vi "Fille Encode.vi"(8 "error in":errorcluster, 11 "Original File":path) -> (2 "string out":string, 10 "Original Data":string)   [LabVIEW 2020]
uses:
  <vilib>/Utility/file.llb/Write Delimited Spreadsheet (string).vi
  <vilib>/Utility/file.llb/Read Delimited Spreadsheet (string).vi
panel:
  out "array":string[][](array[string])
  out "error out":errorcluster
  # "ENCODE"
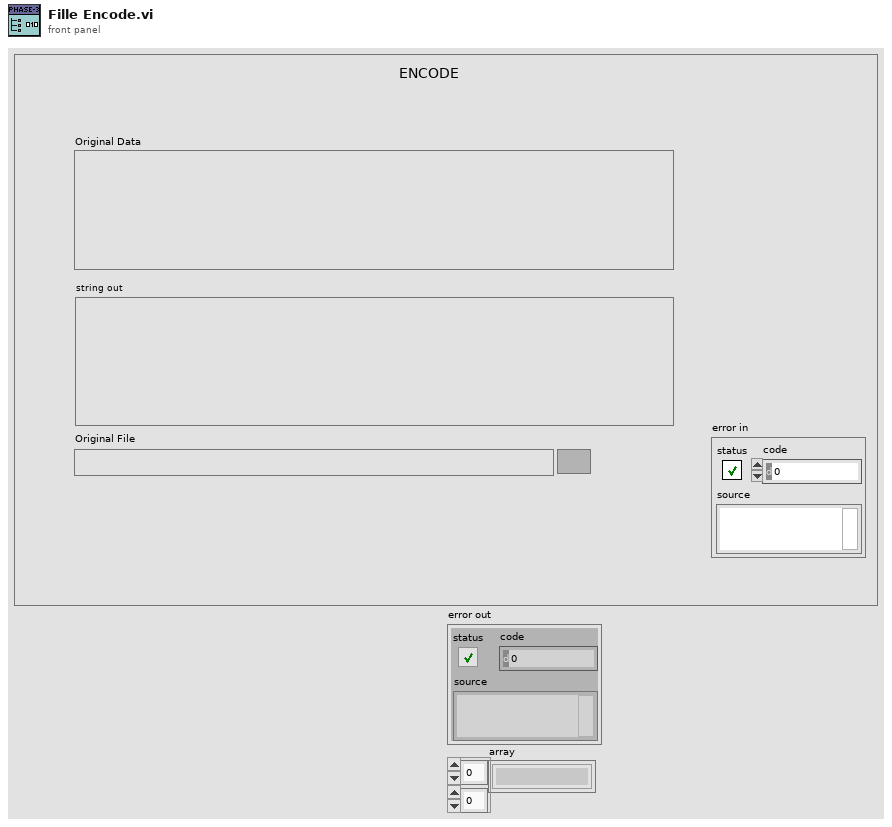
[diagram p1: front panel]
types:
  T1 = cluster{"unsigned byte array[0]":u8, "unsigned byte array[1]":u8, "unsigned byte array[2]":u8}
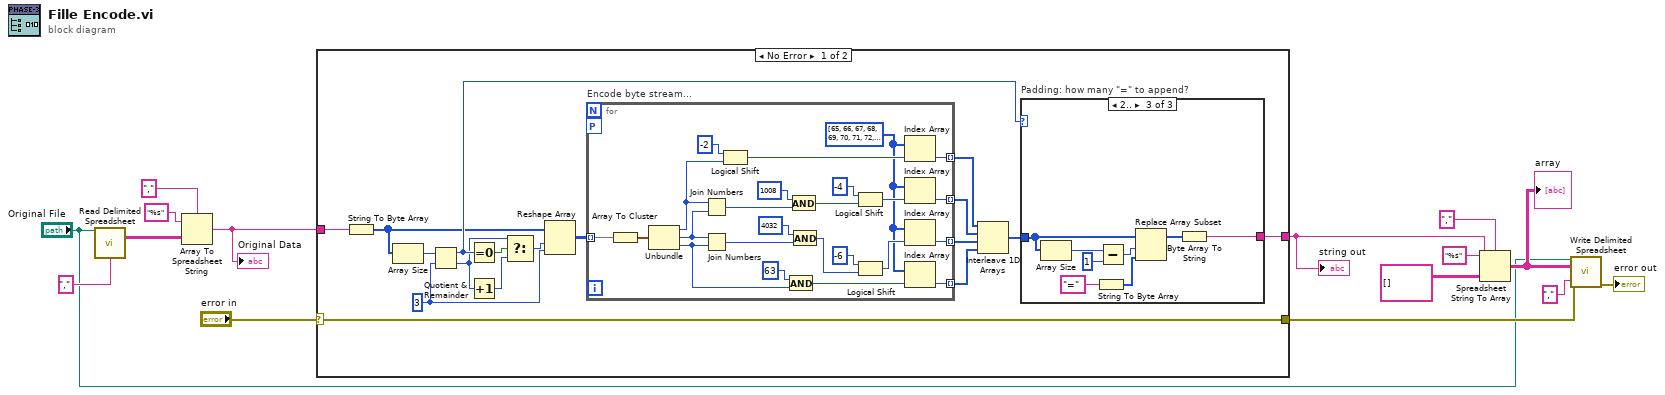
[diagram p0: block diagram]
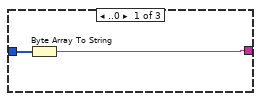
[diagram p2: hidden frame]
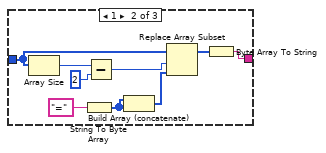
[diagram p3: hidden frame]
diagram:
  n1 = call-poly <vilib>:"Read Delimited Spreadsheet.vi"("file path (dialog if empty)"="Original File", "delimiter (\\t)"="," ("delimiter (\\t)")) -> ("all rows"=w13:string[][])  [unwired: 8 in, 5 out]
  n2 = Array To Spreadsheet String(delimiter (Tab)=",", array=w13, 3:"%s" ("format string")) -> (spreadsheet string=w9:string)
  "Original Data" <- w9
  n3 = case shown="No Error" "error in" {
    selector: "error in" -> [w16 w77]
    tunnel: w9 -> [w19 w76]
    tunnel: [w16 w77] -> w3
    tunnel: [w18 w76] -> w14
    frame No Error {
      w22 = 3 ("y")
      n4 = String To Byte Array(string=w19) -> (unsigned byte array=w23:u8[])
      n5 = Array Size(array=w23) -> (size(s)=w17:i32)
      n6 = Quotient & Remainder(x=w17, y=w22) -> (x-y*floor(x/y)=w31:i32, floor(x/y)=w25:i32)
      n7 = Equal To 0?(x=w31) -> (x = 0?=w32:bool)
      n8 = Increment(x=w25) -> (x+1=w26:i32)
      n9 = Select(t=w25, s=w32, f=w26) -> (s? t:f=w21:i32)
      n10 = Reshape Array(w23, w21, w22) -> (w20:u8[][])
      n11 = for "Encode byte stream..." {
        tunnel: [w35] -> w27 mode=indexing
        tunnel: [w36] -> w28 mode=indexing
        tunnel: [w37] -> w29 mode=indexing
        tunnel: [w38] -> w30 mode=indexing
        workers-P: _ -> [_]
        tunnel: w20 -> [w33] mode=indexing
        w34 = u8[] [65, 66, 67, 68, 69, 70, 71, 72, 73, 74, 75, 76, 77, 78, 79, 80, 81, 82, 83, 84, 85, 86, 87, 88, 89, 90, 97, 98, 99, 100, 101, 102, 103, 104, 105, 106, 107, 108, 109, 110, 111, 112, 113, 114, 115, 116, 117, 118, 119, 120, 121, 122, 48, 49, 50, 51, 52, 53, 54, 55, 56, 57, 43, 47] ("unsigned byte array")
        n12 = Array To Cluster(array=w33) -> (cluster=w56:T1)
        n13 = Unbundle(w56) -> ("unsigned byte array[0]"=w45:u8, "unsigned byte array[1]"=w50:u8, "unsigned byte array[2]"=w44:u8)
        n14 = Join Numbers(hi=w45, lo=w50) -> ((hi.lo)=w54:u16)
        n15 = Join Numbers(hi=w50, lo=w44) -> ((hi.lo)=w49:u16)
        n16 = Logical Shift(y=i8 -2, x=w45) -> (x << y=w42:u8)
        n17 = And(x=u8 63, y=w44) -> (x .and. y?=w39:u8)
        n18 = And(x=u16 1008, y=w54) -> (x .and. y?=w52:u16)
        n19 = And(x=u16 4032, y=w49) -> (x .and. y?=w47:u16)
        n20 = Logical Shift(y=i8 -4, x=w52) -> (x << y=w41:u16)
        n21 = Logical Shift(y=i8 -6, x=w47) -> (x << y=w40:u16)
        n22 = Index Array(array=w34, index=w42) -> (element=w38:u8)
        n23 = Index Array(array=w34, index=w41) -> (element=w37:u8)
        n24 = Index Array(array=w34, index=w40) -> (element=w36:u8)
        n25 = Index Array(array=w34, index=w39) -> (element=w35:u8)
      }
      n26 = Interleave 1D Arrays(w30, w29, w28, w27) -> (w24:u8[])
      n27 = case "Padding: how many \"=\" to append?" shown="2.." w31 {
        tunnel: [w57 w64 w72] -> w18
        tunnel: w24 -> [w58 w62 w70]
        frame ..0 {
          n28 = Byte Array To String(unsigned byte array=w58) -> (string=w57:string)
        }
        frame 1 {
          n29 = Array Size(array=w62) -> (size(s)=w63:i32)
          n30 = String To Byte Array(string="=") -> (unsigned byte array=w60:u8[])
          n31 = Subtract(x=w63, y=2) -> (x-y=w66:i32)
          n32 = Build Array (concatenate)(w60, w60) -> (w59:u8[])
          n33 = Replace Array Subset(array=w62, new element=w59, index=w66) -> (w65:u8[])
          n34 = Byte Array To String(unsigned byte array=w65) -> (string=w64:string)
        }
        frame 2.. {
          n35 = Array Size(array=w70) -> (size(s)=w71:i32)
          n36 = String To Byte Array(string="=") -> (unsigned byte array=w68:u8[])
          n37 = Subtract(x=w71, y=1) -> (x-y=w74:i32)
          n38 = Replace Array Subset(array=w70, new element=w68, index=w74) -> (w73:u8[])
          n39 = Byte Array To String(unsigned byte array=w73) -> (string=w72:string)
        }
      }
    }
    frame Error {
    }
  }
  "string out" <- w14
  n40 = Spreadsheet String To Array(delimiter (Tab)=",", format string="%s", spreadsheet string=w14, array type (2D Dbl)=string[][] [] ("all rows")) -> (array=w6:string[][])
  "array" <- w6
  n41 = call-poly <vilib>:"Write Delimited Spreadsheet.vi"("file path (dialog if empty)"="Original File", "2D data"=w6, "error in (no error)"=w3, "delimiter (\\t)"="," ("delimiter (\\t)")) -> ("error out"=→"error out":errorcluster)  [unwired: 10 in, 1 out]
